vi "Delete Old PPLs From Includes Folder.vi"(8 "error in":errorcluster, 11 "custom device path":path) -> (0 "error out":errorcluster, 3 "custom device path out":path)   [LabVIEW 2020, in "Template Tool.lvlib"]
uses:
  Template Tool.lvlib
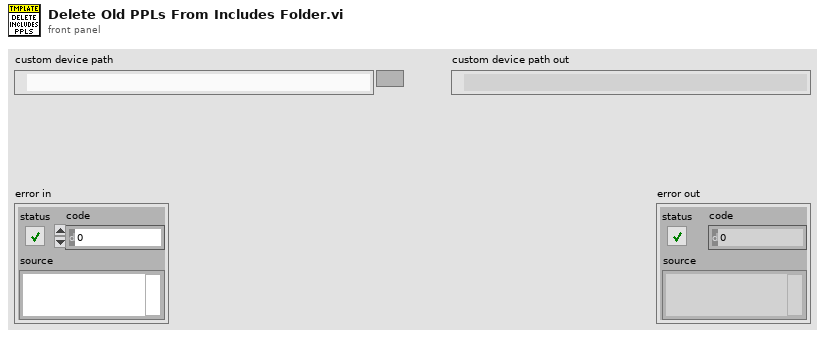
[diagram p1: front panel]
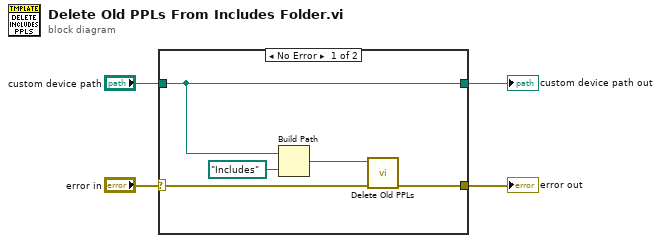
[diagram p0: block diagram]
diagram:
  n1 = case shown="No Error" "error in" {
    selector: "error in" -> [w7 w10]
    tunnel: "custom device path" -> [w8 w11]
    tunnel: [w6 w10] -> w3
    tunnel: [w8 w11] -> w2
    frame No Error {
      n2 = Build Path(base path=w8, name or relative path=path "Includes") -> (appended path=w5:path)
      n3 = call "Delete Old PPLs.vi"("error in"=w7, "PPLs folder path"=w5) -> ("error out"=w6:errorcluster)  [unwired: 9 in]
    }
    frame Error {
    }
  }
  "error out" <- w3
  "custom device path out" <- w2
